vi "Cost.vi"(8 "error in (no error)":errorcluster, 11 "Mocha in":refnum<class "Mocha.lvclass">) -> (0 "error out":errorcluster, 2 "Cost":dbl, 3 "Mocha out":refnum<class "Mocha.lvclass">)   [LabVIEW 2013, in "Mocha.lvclass"]
uses:
  Mocha.lvclass
  Condiment Decorator/Condiment Decorator.lvclass
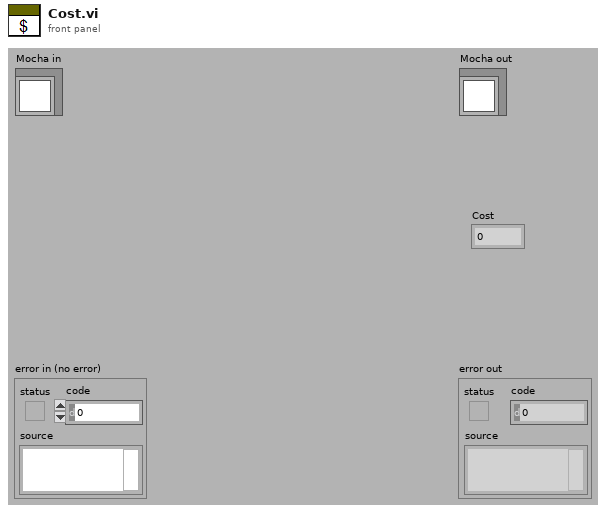
[diagram p1: front panel]
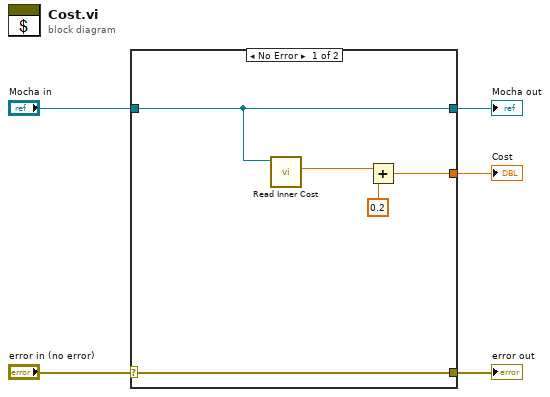
[diagram p0: block diagram]
diagram:
  n1 = case shown="No Error" "error in (no error)" {
    selector: "error in (no error)" -> [w6 w12]
    tunnel: [w6 w12] -> w4
    tunnel: [w8 w11] -> w2
    tunnel: "Mocha in" -> [w8 w11]
    tunnel: [w9 _] -> w1
    frame No Error {
      n2 = call "Read Inner Cost.vi"("Condiment Decorator in"=w8) -> ("Cost"=w7:dbl)  [unwired: 10 in]
      n3 = Add(x=w7, y=0.2) -> (x+y=w9:dbl)
    }
    frame Error {
    }
  }
  "error out" <- w4
  "Mocha out" <- w2
  "Cost" <- w1
